vi "_generate Event.vi"(8 "error in":errorcluster, 10 "event":T1, 11 "VariantBuffer":refnum<class "VariantBuffer.lvclass">) -> (0 "error out":errorcluster, 3 "VariantBuffer out":refnum<class "VariantBuffer.lvclass">)   [LabVIEW 2013, in "CircularBuffer.lvlib" / "VariantBuffer.lvclass"]
uses:
  VariantBuffer.lvclass
  buffer-event -- enum.ctl
  VariantBuffer.lvclass/VariantBuffer.ctl
  buffer-errors -- ring.ctl
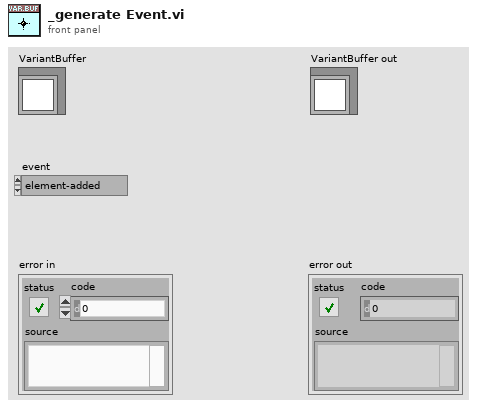
[diagram p1: front panel]
types:
  T1 = typedef "CircularBuffer.lvlib/VariantBuffer.lvclass/buffer-event -- enum.ctl" = enum16{"element-added", "element-removed", "filled", "emptied", "resized", "default-changed", "destroyed"}
  T2 = typedef "CircularBuffer.lvlib/VariantBuffer.lvclass/buffer-errors -- ring.ctl" = i32
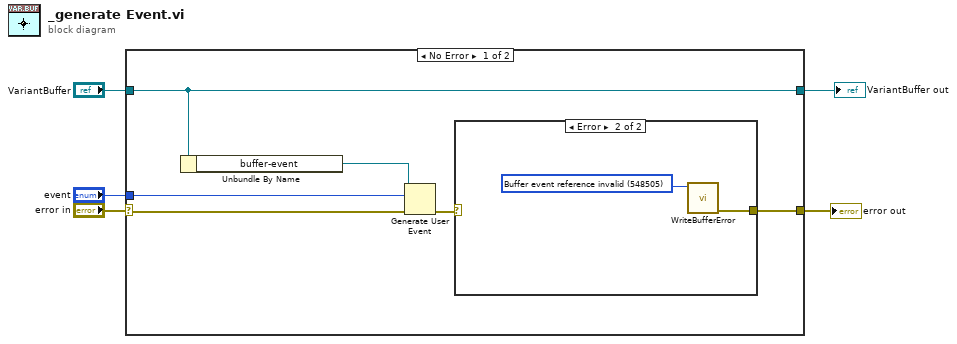
[diagram p0: block diagram]
diagram:
  n1 = case shown="No Error" "error in" {
    selector: "error in" -> [w6 w15]
    tunnel: "event" -> [w11 _]
    tunnel: [w9 w15] -> w4
    tunnel: "VariantBuffer" -> [w7 w16]
    tunnel: [w7 w16] -> w1
    frame No Error {
      n2 = Unbundle By Name(w7) -> ("buffer-event"=w8:refnum<user-event>)
      n3 = Generate User Event(user event=w8, event data cluster=w11, error in=w6) -> (error out=w10:errorcluster)  [unwired: 1 in, 1 out]
      n4 = case shown="Error" w10 {
        selector: w10 -> [w12 _]
        tunnel: [w12 w14] -> w9
        frame No Error {
        }
        frame Error {
          w13 = T2 548505 items=["No error"=0, "Generic Buffer error"=548500, "Buffer is full"=548501, "Buffer is empty"=548502, "Buffer size cannot be 0"=548503, "Buffer reference is invalid"=548504, "Buffer event reference invalid"=548505] ("buffer-errors")
          n5 = call "WriteBufferError.vi"("buffer-errors"=w13) -> ("error out"=w14:errorcluster)  [unwired: 10 in]
        }
      }
    }
    frame Error {
    }
  }
  "error out" <- w4
  "VariantBuffer out" <- w1
